vi "Array Filter.vi"(10 "Input Array 2":dbl[](array[numeric]), 11 "Input Array":dbl[](array[numeric])) -> (2 "Output Array 2":dbl[](array[numeric]), 3 "Output Array":dbl[](array[numeric]))   [LabVIEW 2017]
panel:
  # "Filters the array to values where the value in the second array is nonzero"
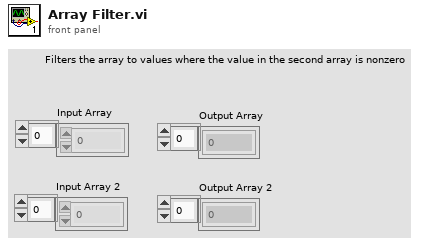
[diagram p1: front panel]
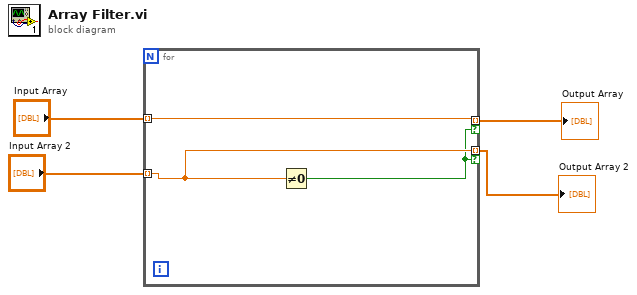
[diagram p0: block diagram]
diagram:
  n1 = for {
    tunnel: "Input Array" -> [w6] mode=indexing
    tunnel: "Input Array 2" -> [w7] mode=indexing
    tunnel: [w7] -> w1 mode=indexing if=w5
    tunnel: [w6] -> w2 mode=indexing if=w5
    n2 = Not Equal To 0?(x=w7) -> (x != 0?=w5:bool)
  }
  "Output Array" <- w2
  "Output Array 2" <- w1
